vi "LOC subConvertArrayOfStringsToStringList.vi"(1 "InputArray":string[](array[string])) -> (0 "OutputString":string)   [LabVIEW 2020, in "Localization_Tools.lvlib"]
uses:
  Localization_Tools.lvlib
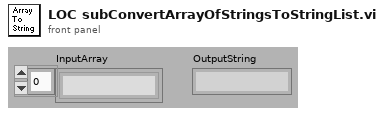
[diagram p1: front panel]
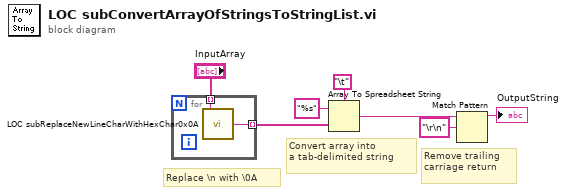
[diagram p0: block diagram]
diagram:
  # "Replace \\n with \\0A"
  # "Convert array into\na tab-delimited string"
  # "Remove trailing\ncarriage return"
  n1 = for {
    tunnel: "InputArray" -> [w9] mode=indexing
    tunnel: [w8] -> w3 mode=indexing
    n2 = call "LOC subReplaceNewLineCharWithHexChar0x0A.vi"("InputString"=w9) -> ("OutputString"=w8:string)
  }
  n3 = Array To Spreadsheet String(delimiter (Tab)="\t", array=w3, 3:"%s" ("format string")) -> (spreadsheet string=w5:string)
  n4 = Match Pattern(string=w5, regular expression="\r\n") -> (before substring=→"OutputString":string)  [unwired: 1 in, 3 out]
